vi "serialize.vi"() -> ()   [LabVIEW 2013, in "tag bus tests.lvlib"]
uses:
  tag bus tests.lvlib
  tag/tag descriptor.lvclass
  tag/tag descriptor.lvclass/tag descriptor.ctl
panel:
  out "ok":bool
  out "Array":bool[](array[boolean])
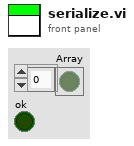
[diagram p1: front panel]
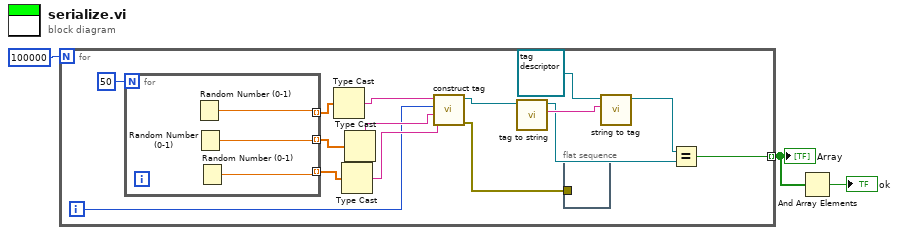
[diagram p0: block diagram]
diagram:
  n1 = for {
    N: 100000 -> [_]
    tunnel: [w5] -> w2 mode=indexing
    i -> [w11]
    n2 = for {
      N: 50 -> [_]
      tunnel: [w21] -> w16 mode=indexing
      tunnel: [w20] -> w17 mode=indexing
      tunnel: [w19] -> w15 mode=indexing
      n3 = Random Number (0-1)() -> (number: 0 to 1=w20:dbl)
      n4 = Random Number (0-1)() -> (number: 0 to 1=w21:dbl)
      n5 = Random Number (0-1)() -> (number: 0 to 1=w19:dbl)
    }
    n6 = Type Cast(x=w17) -> (*(type *) &x=w14:string)  [unwired: 1 in]
    n7 = Type Cast(x=w15) -> (*(type *) &x=w12:string)  [unwired: 1 in]
    n8 = Type Cast(x=w16) -> (*(type *) &x=w13:string)  [unwired: 1 in]
    n9 = call "construct tag.vi"("raw default"=w12, "metadata"=w13, "data type"=w11, "name"=w14) -> ("error out"=w4:errorcluster, "system tag out"=w10:refnum<class "tag descriptor.lvclass">)  [unwired: 6 in]
    n10 = call "tag to string.vi"("tag descriptor in"=w10) -> ("tag string"=w9:string, "tag descriptor out"=w6:refnum<class "tag descriptor.lvclass">)  [unwired: 8 in, 1 out]
    n11 = flat-sequence {
      tunnel: w4 -> [_]
      frame #0 {
      }
    }
    n12 = call "string to tag.vi"("tag string"=w9, "tag descriptor in"=refnum<class "tag descriptor.lvclass"> refnum) -> ("tag descriptor out"=w7:refnum<class "tag descriptor.lvclass">)  [unwired: 8 in, 1 out]
    n13 = Equal?(x=w7, y=w6) -> (x = y?=w5:bool)
  }
  "Array" <- w2
  n14 = And Array Elements(Boolean array=w2) -> (logical AND=→"ok":bool)
